vi "InsertItem.vi"(7 "Parent Tag":string, 8 "error in (no error)":errorcluster, 10 "MenuItem":refnum<class "MGI_MenuItem.lvclass">, 11 "MenuStrip in":refnum<class "MGI_MenuStrip.lvclass">) -> (0 "error out":errorcluster, 3 "MenuStrip out":refnum<class "MGI_MenuStrip.lvclass">)   [LabVIEW 2016, in "MGI_MenuStrip.lvclass"]
doc: "Inserts a menu item into the menu.\n\nAuthored by Derek E. Trepanier\nsupport@mooregoodideas.com\nwww.mooregoodideas.com\n\nCopyright (c) 2012, Moore Good Ideas, Inc.\n\nAll rights reserved.\n\nRedistribution and use in source and binary forms, with or without modification, are permitted provided that the following conditions are met:\n\n * Redistributions of source code must retain the above copyright notice, this list of conditions and the following disclaimer.\n * Redistributions in binary form must reproduce the above copyright notice, this list of conditions and the following disclaimer in the documentation and/or other materials provided with the distribution.\n * Neither the name of Moore Good Ideas, Inc. nor the names of its contributors may be used to endorse or promote products derived from this software without specific prior written permission.\n\nTHIS SOFTWARE IS PROVIDED BY THE COPYRIGHT HOLDERS AND CONTRIBUTORS \"AS IS\" AND ANY EXPRESS OR IMPLIED WARRANTIES, INCLUDING, BUT NOT LIMITED TO, THE IMPLIED WARRANTIES OF MERCHANTABILITY AND FITNESS FOR A PARTICULAR PURPOSE ARE DISCLAIMED. IN NO EVENT SHALL THE COPYRIGHT OWNER OR CONTRIBUTORS BE LIABLE FOR ANY DIRECT, INDIRECT, INCIDENTAL, SPECIAL, EXEMPLARY, OR CONSEQUENTIAL DAMAGES (INCLUDING, BUT NOT LIMITED TO, PROCUREMENT OF SUBSTITUTE GOODS OR SERVICES; LOSS OF USE, DATA, OR PROFITS; OR BUSINESS INTERRUPTION) HOWEVER CAUSED AND ON ANY THEORY OF LIABILITY, WHETHER IN CONTRACT, STRICT LIABILITY, OR TORT (INCLUDING NEGLIGENCE OR OTHERWISE) ARISING IN ANY WAY OUT OF THE USE OF THIS SOFTWARE, EVEN IF ADVISED OF THE POSSIBILITY OF SUCH DAMAGE."
uses:
  <userlib>/_MGI/Menu Building/MenuTypes/MenuStrip/MGI_MenuStrip.lvclass
  <userlib>/_MGI/Menu Building/MenuItem/MGI_MenuItem.lvclass
  <userlib>/_MGI/Menu Building/MenuTypes/MenuStrip/MGI_MenuStrip.lvclass/MGI_MenuStrip.ctl
  System.Windows.Forms
  <userlib>/_MGI/Menu Building/MenuItem/Read Enabled.vi
  <userlib>/_MGI/Menu Building/MenuItem/Read Checked.vi
  <userlib>/_MGI/Menu Building/MenuItem/Read Full Tag.vi
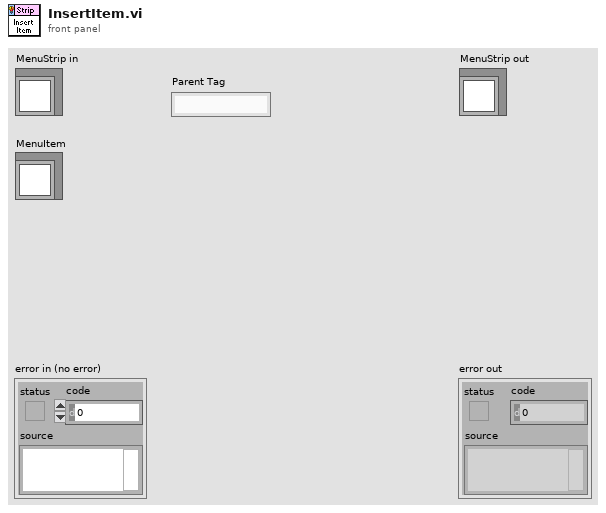
[diagram p1: front panel]
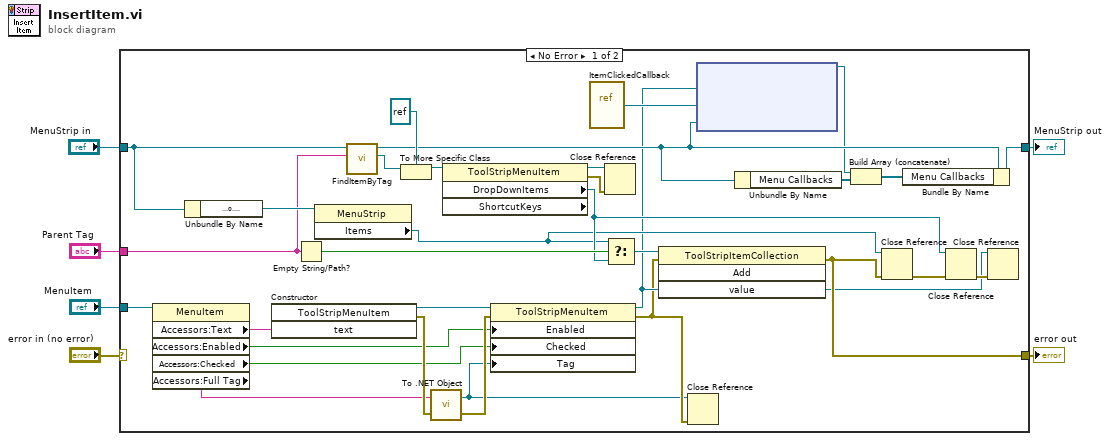
[diagram p0: block diagram]
diagram:
  n1 = case shown="No Error" "error in (no error)" {
    selector: "error in (no error)" -> [_ w40]
    tunnel: [w16 w40] -> w5
    tunnel: [w24 w39] -> w4
    tunnel: "MenuStrip in" -> [w30 w39]
    tunnel: "MenuItem" -> [w38 _]
    tunnel: "Parent Tag" -> [w29 _]
    frame No Error {
      n2 = property class="MenuItem"(reference=w38) -> ("Accessors:Text"=w37:string, "Accessors:Enabled"=w8:bool, "Accessors:Checked"=w7:bool, "Accessors:Full Tag"=w19:string)  [unwired: 1 in, 2 out]
      n3 = Unbundle By Name(w30) -> ("MenuStrip"=w35:refnum<k24>)
      n4 = constructor class="ToolStripMenuItem"("text"=w37) -> (reference out=w36:refnum<k24>, error out=w32:errorcluster)  [unwired: 3 in, 2 out]
      n5 = Empty String/Path?(string/path=w29) -> (empty?=w34:bool)
      n6 = property class="MenuStrip"(reference=w35) -> ("Items"=w17:refnum<k24>)  [unwired: 1 in, 2 out]
      n7 = call <userlib>:"FindItemByTag.vi"("Tag"=w29, "MenuStrip in"=w30) -> ("Tool Strip Menu Item"=w27:refnum<k24>, "MenuStrip out"=w25:refnum<class "MGI_MenuStrip.lvclass">)  [unwired: 7 in, 1 out]
      n8 = To More Specific Class(target class=refnum<k24> refnum ("new reference"), reference=w27) -> (specific class reference=w26:refnum<k24>)  [unwired: 1 in, 1 out]
      n9 = call <vilib>:"To .NET Object.vi"("error in (no error)"=w32, "anything"=w19) -> ("error out"=w31:errorcluster, ".NET object"=w9:refnum<k24>)
      n10 = property class="ToolStripMenuItem" props=["DropDownItems", "ShortcutKeys"](reference=w26) -> (reference out=w11:refnum<k24>, error out=w12:errorcluster, "DropDownItems"=w18:refnum<k24>)  [unwired: 1 in, 1 out]
      n11 = property class="ToolStripMenuItem"(reference=w36, error in=w31, "Enabled"=w8, "Checked"=w7, "Tag"=w9) -> (reference out=w13:refnum<k24>, error out=w10:errorcluster)
      n12 = vi-ref <userlib>:"ItemClickedCallback.vi"() -> ("vi reference"=w20:refnum<vi>)
      n13 = Close Reference(reference=w11, error in (no error)=w12) -> ()  [unwired: 1 out]
      n14 = Select(t=w17, s=w34, f=w18) -> (s? t:f=w33:refnum<k24>)
      n15 = invoke class="ToolStripItemCollection" method="Add"(reference=w33, error in=w10, "value"=w13) -> (error out=w16:errorcluster)  [unwired: 1 in, 3 out]
      n16 = Close Reference(reference=w9, error in (no error)=w10) -> ()  [unwired: 1 out]
      n17 = node(w13, w20, w25) -> (w21:refnum<k27>)  [unwired: 2 in, 1 out]
      n18 = Unbundle By Name(w25) -> ("Menu Callbacks"=w23:refnum<k27>[])
      n19 = Build Array (concatenate)(w21, w23) -> (w22:refnum<k27>[])
      n20 = Close Reference(reference=w17, error in (no error)=w16) -> (error out=w15:errorcluster)
      n21 = Bundle By Name(cluster=w25, "Menu Callbacks"=w22) -> (w24:refnum<class "MGI_MenuStrip.lvclass">)
      n22 = Close Reference(reference=w18, error in (no error)=w15) -> (error out=w14:errorcluster)
      n23 = Close Reference(reference=w13, error in (no error)=w14) -> ()  [unwired: 1 out]
    }
    frame Error {
    }
  }
  "error out" <- w5
  "MenuStrip out" <- w4
